vi "Wait for Work Command.vi"(8 "error in (no error)":errorcluster, 9 "timeout in ms (5000)":i32=5000 format="%d ms", 11 "Dispatcher in":refnum<class "Dispatcher.lvclass">) -> (0 "error out":errorcluster, 1 "timed out?":bool, 2 "command":T1, 3 "Dispatcher out":refnum<class "Dispatcher.lvclass">)   [LabVIEW 2017, in "DSF Core.lvlib" / "Dispatcher.lvclass"]
uses:
  Dispatcher.lvclass
  Interfaces/Dispatcher/Command Data.ctl
  Interfaces/Dispatcher/Command.ctl
  Interfaces/Dispatcher/Parameters.ctl
  Dispatcher.lvclass/Dispatcher.ctl
  Interfaces/Dispatcher/Dispatcher Interface.lvclass
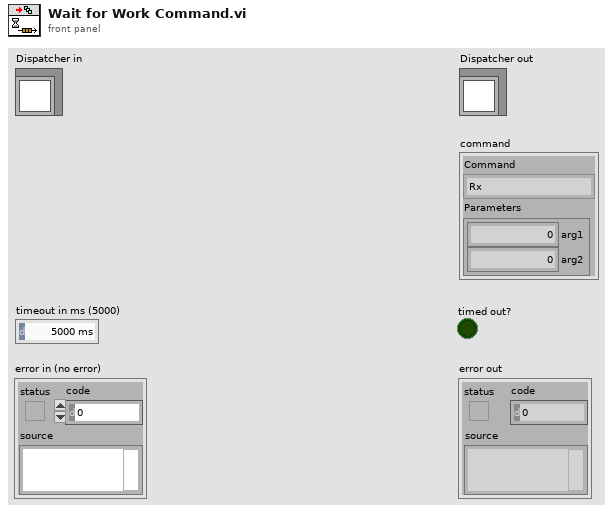
[diagram p1: front panel]
types:
  T1 = typedef "DSF Core.lvlib/Dispatcher Interface.lvclass/Command Data.ctl" = cluster{"Command":T2, "Parameters":T3}
  T2 = typedef "DSF Core.lvlib/Dispatcher Interface.lvclass/Command.ctl" = enum8{"Rx", "Tx", "Shutdown"}
  T3 = typedef "DSF Core.lvlib/Dispatcher Interface.lvclass/Parameters.ctl" = cluster{"arg1":u64, "arg2":u64}
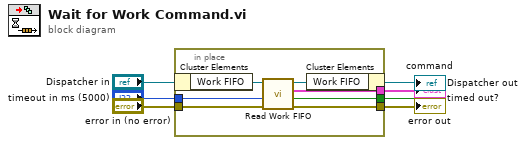
[diagram p0: block diagram]
diagram:
  n1 = in-place {
    in-place-border: "timeout in ms (5000)" -> [w14]
    in-place-border: "error in (no error)" -> [w13]
    in-place-border: [w12] -> w3
    in-place-border: [w11] -> w2
    in-place-border: [w8] -> w1
    n2 = in-place-cluster #1("Dispatcher in") -> ("Work FIFO"=w10:refnum<k33>)
    n3 = call "Read Work FIFO.vi"("error in (no error)"=w13, "timeout in ms (0)"=w14, "Work FIFO in"=w10) -> ("error out"=w12:errorcluster, "timed out?"=w8:bool, "command"=w11:T1, "Work FIFO out"=w9:refnum<k33>)  [unwired: 4 in, 1 out]
    n4 = in-place-cluster #1("Work FIFO"=w9) -> (→"Dispatcher out":refnum<class "Dispatcher.lvclass">)
  }
  "error out" <- w3
  "command" <- w2
  "timed out?" <- w1
